vi "SetCtComm.vi"(1 "ConnectID":u32) -> ()   [LabVIEW 2011]
uses:
  Globals/SysGlbs.vi
  Globals/DCfgGlbs.vi
  Globals/CTCGlbs.vi
  Windows/System32/Ctccom32v2.dll
panel:
  out "Err Msg":string
  out "Err":bool
  in  "Timeout (ms)":u32=250
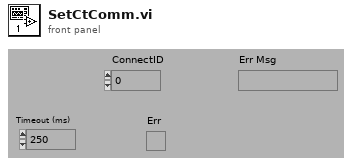
[diagram p1: front panel]
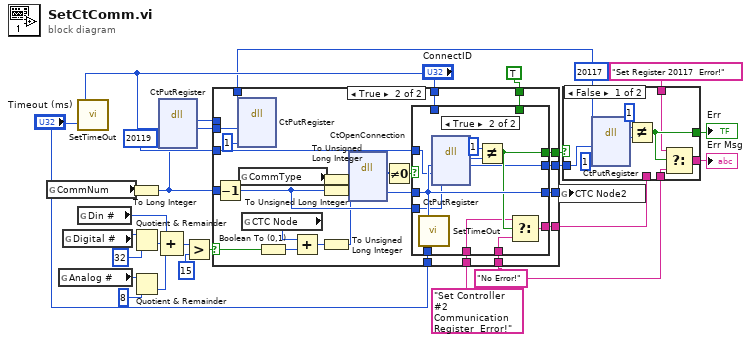
[diagram p0: block diagram]
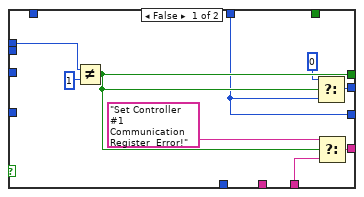
[diagram p3: hidden frame]
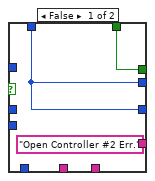
[diagram p4: hidden frame]
diagram:
  w1 = u32 20117
  w12 = "No Error!"
  w15 = u32 20119
  n1 = global read "CTCGlbs.vi" "CommNum"() -> (w16:i16)
  n2 = global read "SysGlbs.vi" "Analog #"() -> (w24:u32)
  n3 = global read "SysGlbs.vi" "Digital #"() -> (w28:u32)
  n4 = call "SetTimeOut.vi"("ConnectID"="ConnectID", "Timeout (ms)"="Timeout (ms)") -> ()  [unwired: 3 out]
  n5 = global read "DCfgGlbs.vi" "Din #"() -> (w25:i32)
  n6 = To Long Integer(number=w16) -> (32bit integer=w4:i32)
  n7 = Quotient & Remainder(x=w28, y=u32 32) -> (floor(x/y)=w26:u32)  [unwired: 1 out]
  n8 = Quotient & Remainder(x=w24, y=u32 8) -> (floor(x/y)=w22:u32)  [unwired: 1 out]
  n9 = dll-call lib="C:/WINNT/system32/CtcEmcorev2.dll" fn="CtPutRegister"("ConnectID"="ConnectID", "Register"=w15, "pValue"=w4) -> (w13:u32, "ConnectID"=w2:u32)  [unwired: 5 in, 2 out]
  n10 = Compound Arithmetic op=ADD(w25, w26, w22) -> (w21:u32)
  n11 = Greater?(x=w21, y=15) -> (0:w18:bool)
  n12 = case shown="True" w18 {
    selector: w18 -> [_ w60]
    tunnel: "ConnectID" -> [w31 w58]
    tunnel: [w31 w57] -> w19
    tunnel: w4 -> [_ w52]
    tunnel: "Timeout (ms)" -> [_ w51]
    tunnel: w15 -> [_ w50]
    tunnel: TRUE -> [_ w49]
    tunnel: [w33 w48] -> w7
    tunnel: [w32 w47] -> w10
    tunnel: w13 -> [w37 _]
    tunnel: w12 -> [w35 w46]
    tunnel: "Set Controller #2 Communication Register  Error!" -> [_ w45]
    tunnel: [w29 w44] -> w9
    tunnel: w2 -> [_ w40]
    tunnel: w1 -> [_ w38]
    frame False {
      n13 = Not Equal?(x=w37, y=u32 1) -> (x != y?=w32:bool)
      n14 = Select(t=u32 0, s=w32, f=w31) -> (s? t:f=w29:u32)
      n15 = Select(t="Set Controller #1 Communication Register  Error!", s=w32, f=w35) -> (s? t:f=w33:string)
    }
    frame True {
      n16 = Decrement(x=w52) -> (x-1=w55:i32)
      n17 = dll-call lib="C:/WINNT/system32/CtcEmcorev2.dll" fn="CtPutRegister"("ConnectID"=w40, "Register"=w38, "pValue"=1) -> ()  [unwired: 7 in, 2 out]
      n18 = global read "CTCGlbs.vi" "CommType"() -> (w62:u16)
      n19 = global read "CTCGlbs.vi" "CTC Node"() -> (w53:i16)
      n20 = Boolean To (0,1)(Boolean=w60) -> (0, 1=w54:i16)
      n21 = Add(x=w53, y=w54) -> (x+y=w59:i16)
      n22 = To Unsigned Long Integer(number=w62) -> (unsigned 32bit integer=w43:u32)
      n23 = To Unsigned Long Integer(number=w55) -> (unsigned 32bit integer=w42:u32)
      n24 = To Unsigned Long Integer(number=w59) -> (unsigned 32bit integer=w41:u32)
      n25 = dll-call lib="C:/WINNT/system32/CtcEmcorev2.dll" fn="CtOpenConnection"("ConnectType"=w43, "LocalAddress"=w42, "RemotAddress"=w41) -> (w56:u32)  [unwired: 6 in, 2 out]
      n26 = Not Equal To 0?(x=w56) -> (x != 0?=w61:bool)
      n27 = case shown="True" w61 {
        tunnel: w58 -> [w63 _]
        tunnel: [w63 w75] -> w57
        tunnel: w56 -> [_ w75]
        tunnel: w55 -> [_ w74]
        tunnel: w51 -> [_ w76]
        tunnel: w50 -> [_ w73]
        tunnel: w49 -> [w64 _]
        tunnel: ["Open Controller #2 Err." w69] -> w48
        tunnel: [w64 w68] -> w47
        tunnel: w46 -> [_ w70]
        tunnel: w45 -> [_ w67]
        tunnel: [w63 w66] -> w44
        frame False {
        }
        frame True {
          n28 = call "SetTimeOut.vi"("ConnectID"=w75, "Timeout (ms)"=w76) -> ()  [unwired: 3 out]
          n29 = dll-call lib="C:/WINNT/system32/CtcEmcorev2.dll" fn="CtPutRegister"("ConnectID"=w75, "Register"=w73, "pValue"=w74) -> (w72:u32, "ConnectID"=w66:u32)  [unwired: 5 in, 2 out]
          n30 = Not Equal?(x=u32 1, y=w72) -> (x != y?=w68:bool)
          n31 = Select(t=w67, s=w68, f=w70) -> (s? t:f=w69:string)
        }
      }
    }
  }
  n32 = global write "CTCGlbs.vi" "CTC Node2"(w19) -> ()
  n33 = case shown="False" w10 {
    selector: w10 -> [_ w87]
    tunnel: w9 -> [w84 _]
    tunnel: [w81 w87] -> w8
    tunnel: w7 -> [_ w86]
    tunnel: [w79 w86] -> w6
    tunnel: w12 -> [w80 _]
    tunnel: "Set Register 20117  Error!" -> [w78 _]
    tunnel: w1 -> [w77 _]
    frame False {
      n34 = dll-call lib="C:/WINNT/system32/CtcEmcorev2.dll" fn="CtPutRegister"("ConnectID"=w84, "Register"=w77, "pValue"=1) -> (w83:u32)  [unwired: 6 in, 2 out]
      n35 = Not Equal?(x=u32 1, y=w83) -> (x != y?=w81:bool)
      n36 = Select(t=w78, s=w81, f=w80) -> (s? t:f=w79:string)
    }
    frame True {
    }
  }
  "Err" <- w8
  "Err Msg" <- w6
